vi "Self Test.vi"(8 "error in":errorcluster, 11 "Acopian in":refnum<class "Acopian.lvclass">) -> (0 "error out":errorcluster, 3 "Acopian out":refnum<class "Acopian.lvclass">)   [LabVIEW 2019, in "Acopian.lvlib" / "Acopian.lvclass"]
uses:
  Library/Acopian.lvclass
  Library/Acopian.lvclass/Acopian.ctl
  builds/Instruments/PowerSupply.lvlibp/Library/PowerSupply.lvclass
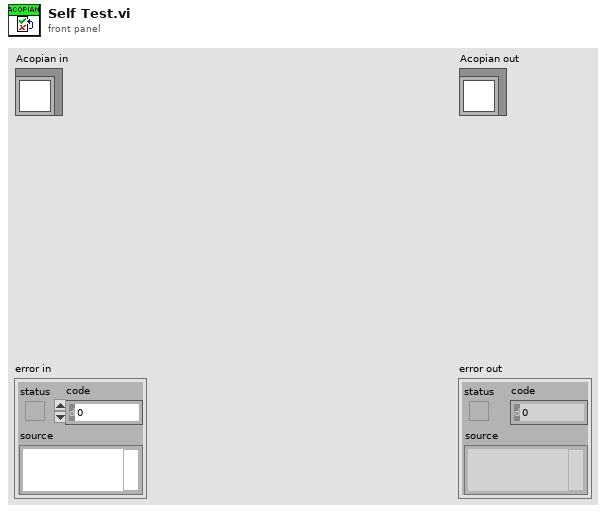
[diagram p1: front panel]
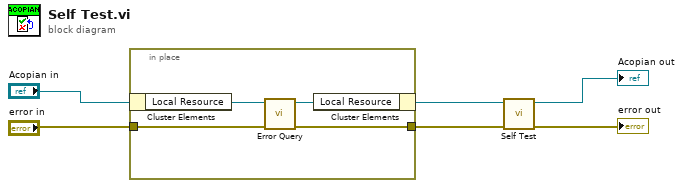
[diagram p0: block diagram]
diagram:
  n1 = in-place {
    in-place-border: [w8] -> w3
    in-place-border: "error in" -> [w7]
    n2 = in-place-cluster #1("Acopian in") -> ("Local Resource"=w10:refnum<visa-resource-name>)
    n3 = call "Error Query.vi"("error in"=w7, "VISA resource in"=w10) -> ("error out"=w8:errorcluster, "VISA resource out"=w9:refnum<visa-resource-name>)  [unwired: 6 in, 2 out]
    n4 = in-place-cluster #1("Local Resource"=w9) -> (w2:refnum<class "Acopian.lvclass">)
  }
  n5 = call-parent "Self Test.vi"("error in"=w3, "Instruments in"=w2) -> ("error out"=→"error out":errorcluster, "Instruments out"=→"Acopian out":refnum<class "Acopian.lvclass">)  [unwired: 8 in]
